vi "Final get list.vi"(4 "Year":i32, 6 "Month":i32, 10 "Dates in in":timestamp[](array[timestamp]), 11 "Instances":string) -> (2 "Dates out":timestamp[](array[timestamp]), 3 "User string":string)   [LabVIEW 2015]
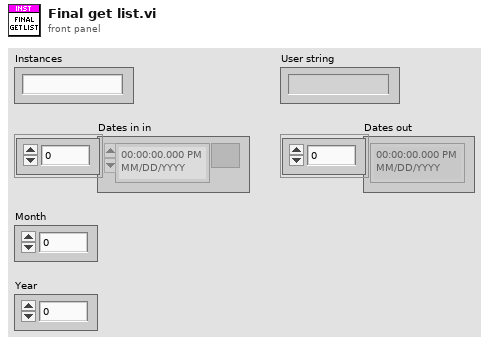
[diagram p1: front panel]
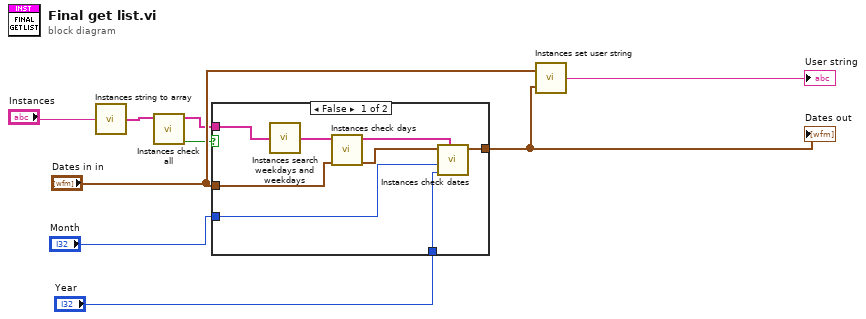
[diagram p0: block diagram]
diagram:
  n1 = call "Instances string to array.vi"("String"="Instances") -> ("Array"=w2:string[])
  n2 = call "Instances check all.vi"("Array in"=w2) -> ("Any all days?"=w3:bool, "Array out"=w4:string[])  [unwired: 9 in]
  n3 = case shown="False" w3 {
    tunnel: w4 -> [w17 _]
    tunnel: "Dates in in" -> [w15 w18]
    tunnel: [w14 w18] -> w6
    tunnel: "Year" -> [w11 _]
    tunnel: "Month" -> [w10 _]
    frame False {
      n4 = call "Instances search weekdays and weekdays.vi"("Array in"=w17) -> ("Array out"=w16:string[])
      n5 = call "Instances check days.vi"("Dates in"=w15, "Array in"=w16) -> ("Dates undelivered"=w13:timestamp[], "Array out"=w12:string[])  [unwired: 8 in]
      n6 = call "Instances check dates.vi"("Array in"=w12, "Year"=w11, "Month"=w10, "Dates undelivered"=w13) -> ("Dates undelivered out"=w14:timestamp[])  [unwired: 6 in]
    }
    frame True {
    }
  }
  "Dates out" <- w6
  n7 = call "Instances set user string.vi"("Dates undelivered in"=w6, "Dates in"="Dates in in") -> ("User string"=→"User string":string)
